vi "Compile project.vi"(8 "error in (no error)":errorcluster, 10 "parameters":T1, 11 "ServiceManager in":refnum<class "ServiceManager.lvclass">) -> (0 "error out":errorcluster, 3 "ServiceManager out":refnum<class "ServiceManager.lvclass">)   [LabVIEW 2012, in "ServiceManager.lvclass"]
uses:
  ServiceManager.lvclass
  boot_parameters_cluster.ctl
  Murmex/LabVIEW/Murmex/Murmex/component_specification_cluster.ctl
  Murmex/LabVIEW/Murmex/Murmex/Murmex.lvclass
panel:
  out "Generated files 2":path[](array[path])
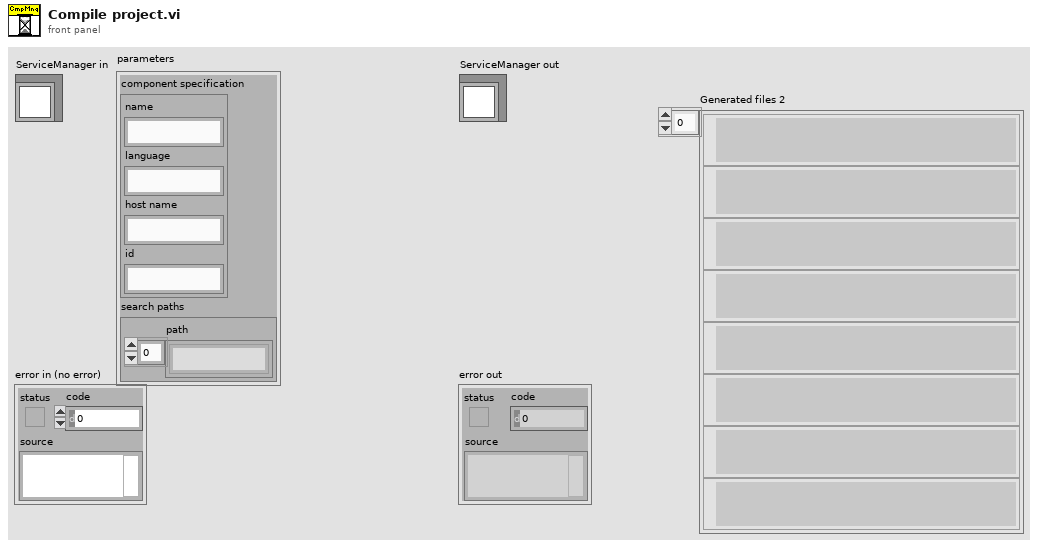
[diagram p1: front panel]
types:
  T1 = typedef "ServiceManager.lvclass/boot_parameters_cluster.ctl" = cluster{"component specification":T2, "search paths":cluster{"path":string[]}}
  T2 = typedef "Murmex.lvlib/Murmex.lvclass/component_specification_cluster.ctl" = cluster{"name":string, "language":string, "host name":string, "id":string}
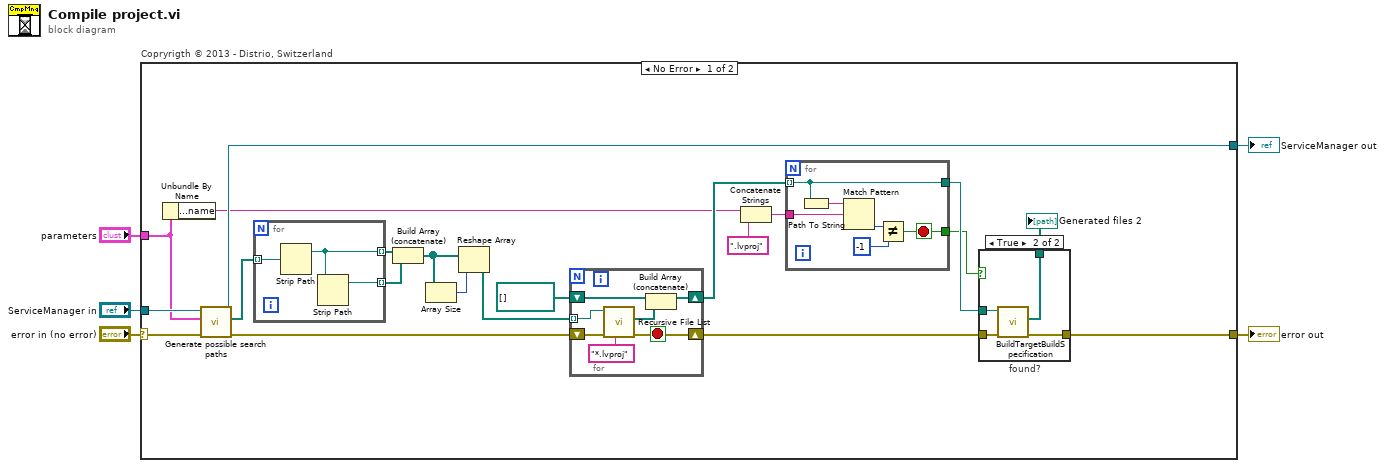
[diagram p0: block diagram]
diagram:
  n1 = case "Copryrigth © 2013 - Distrio, Switzerland" shown="No Error" "error in (no error)" {
    selector: "error in (no error)" -> [w26 w49]
    tunnel: [w15 w49] -> w4
    tunnel: [w24 w48] -> w2
    tunnel: "ServiceManager in" -> [w25 w48]
    tunnel: "parameters" -> [w14 _]
    frame No Error {
      n2 = Unbundle By Name(w14) -> ("component specification.name"=w13:string)
      n3 = call-dynamic "Generate possible search paths.vi"("error in (no error)"=w26, "parameters"=w14, "ServiceManager in"=w25) -> ("error out"=w18:errorcluster, "path array out"=w7:path[], "ServiceManager out"=w24:refnum<class "ServiceManager.lvclass">)  [unwired: 6 in]
      n4 = for {
        tunnel: w7 -> [w29] mode=indexing
        tunnel: [w28] -> w11 mode=indexing
        tunnel: [w27] -> w10 mode=indexing
        n5 = Strip Path(path=w29) -> (stripped path=w28:path)  [unwired: 1 out]
        n6 = Strip Path(path=w28) -> (stripped path=w27:path)  [unwired: 1 out]
      }
      n7 = Build Array (concatenate)(w11, w10) -> (w8:path[])
      n8 = Array Size(array=w8) -> (size(s)=w9:i32)
      n9 = Reshape Array(w8, w9) -> (w6:path[])
      n10 = for {
        tunnel: w6 -> [w40] mode=indexing
        shift-right: [w37] -> w16
        shift-left: path[] [] ("All Files in Dir") -> [w39]
        shift-right: [w35] -> w20
        shift-left: w18 -> [w41]
        stop <- w35 stop-if-true
        n11 = call <vilib>:"Recursive File List.vi"("pattern"="*.lvproj" ("string"), "error in (no error)"=w41, "Folder Path"=w40) -> ("error out"=w35:errorcluster, "All Files in Dir"=w38:path[])  [unwired: 4 in, 3 out]
        n12 = Build Array (concatenate)(w39, w38) -> (w37:path[])
      }
      n13 = Concatenate Strings(w13, ".lvproj" ("string")) -> (w22:string)
      n14 = for {
        tunnel: w16 -> [w42] mode=indexing
        tunnel: w22 -> [w46]
        tunnel: [w43] -> w12
        tunnel: [w42] -> w21
        stop <- w43 stop-if-true
        n15 = Path To String(path=w42) -> (string=w47:string)
        n16 = Match Pattern(string=w47, regular expression=w46) -> (offset past match=w45:i32)  [unwired: 1 in, 3 out]
        n17 = Not Equal?(x=w45, y=-1) -> (x != y?=w43:bool)
      }
      n18 = case "found?" shown="True" w12 {
        tunnel: w21 -> [_ w34]
        tunnel: w20 -> [w30 w33]
        tunnel: [_ w32] -> w19
        tunnel: [w30 w31] -> w15
        frame False {
        }
        frame True {
          n19 = call <vilib>:"BuildTargetBuildSpecification.vi"("error in (no error)"=w33, "Path to project"=w34) -> ("error out"=w31:errorcluster, "Generated files"=w32:path[])  [unwired: 8 in]
        }
      }
      "Generated files 2" <- w19
    }
    frame Error {
    }
  }
  "error out" <- w4
  "ServiceManager out" <- w2
